vi "attributes-identity-test.vi"(8 "error in (no error)":errorcluster) -> (0 "error out":errorcluster)   [LabVIEW 2013]
uses:
  src/Support/Attribute.Identity/Attribute.Identity.lvclass/Attribute.Identity.ctl
  src/Support/Attribute/Attribute.lvclass/Attribute.ctl
  <vilib>/Utility/LVClass/Get LV Class Name.vi
  <vilib>/addons/_JKI Toolkits/Caraya/classes/Test/Test.lvclass
  <vilib>/addons/_JKI Toolkits/Caraya/classes/Assert/Assert.lvclass
  src/Support/Attribute.Identity/Attribute.Identity.lvclass
  src/Support/Attribute/Attribute.lvclass
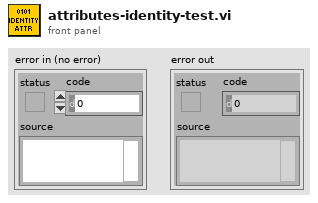
[diagram p1: front panel]
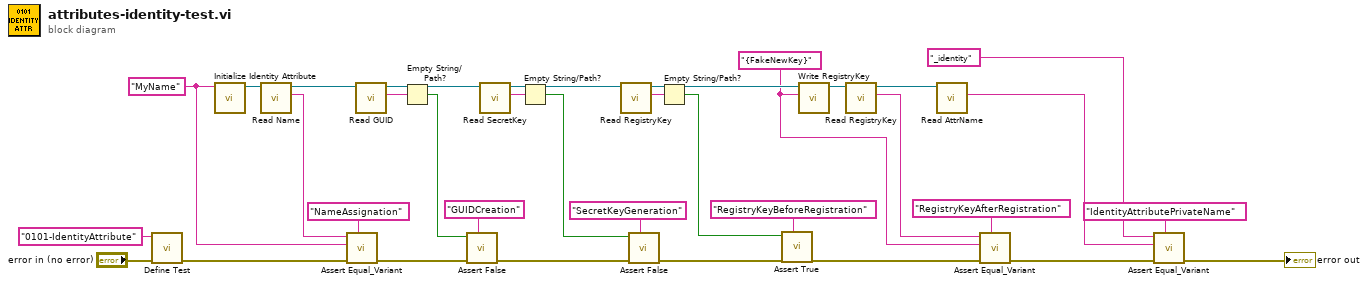
[diagram p0: block diagram]
diagram:
  w8 = "{FakeNewKey}" ("Label (VI Title)")
  w25 = "MyName" ("Name")
  n1 = call <vilib>:"Define Test.vi"("error in (no error)"="error in (no error)", "Label (VI Title)"="0101-IdentityAttribute") -> ("error out"=w33:errorcluster)  [unwired: 9 in]
  n2 = call "Initialize Identity Attribute.vi"("Given Name"=w25) -> ("Attribute.Identity"=w30:refnum<class "Attribute.Identity.lvclass">)  [unwired: 9 in, 1 out]
  n3 = call "Read Name.vi"("Attribute.Identity in"=w30) -> ("Name"=w26:string, "Attribute.Identity out"=w29:refnum<class "Attribute.Identity.lvclass">)  [unwired: 8 in, 1 out]
  n4 = call <vilib>:"Assert Equal_Variant.vi"("Label"="NameAssignation" ("Label (VI Title)"), "error in (no error)"=w33, "Y"=w25, "X"=w26) -> ("error out"=w23:errorcluster)  [unwired: 7 in]
  n5 = call "Read GUID.vi"("Attribute.Identity in"=w29) -> ("GUID"=w24:string, "Attribute.Identity out"=w28:refnum<class "Attribute.Identity.lvclass">)  [unwired: 8 in, 1 out]
  n6 = Empty String/Path?(string/path=w24) -> (empty?=w22:bool)
  n7 = call <vilib>:"Assert False.vi"("Label"="GUIDCreation" ("Label (VI Title)"), "error in (no error)"=w23, "False?"=w22) -> ("error out"=w20:errorcluster)  [unwired: 8 in]
  n8 = call "Read SecretKey.vi"("Attribute.Identity in"=w28) -> ("SecretKey"=w18:string, "Attribute.Identity out"=w16:refnum<class "Attribute.Identity.lvclass">)  [unwired: 8 in, 1 out]
  n9 = Empty String/Path?(string/path=w18) -> (empty?=w17:bool)
  n10 = call "Read RegistryKey.vi"("Attribute.Identity in"=w16) -> ("RegistryKey"=w14:string, "Attribute.Identity out"=w15:refnum<class "Attribute.Identity.lvclass">)  [unwired: 8 in, 1 out]
  n11 = call <vilib>:"Assert False.vi"("Label"="SecretKeyGeneration" ("Label (VI Title)"), "error in (no error)"=w20, "False?"=w17) -> ("error out"=w12:errorcluster)  [unwired: 8 in]
  n12 = Empty String/Path?(string/path=w14) -> (empty?=w11:bool)
  n13 = call <vilib>:"Assert True.vi"("Label"="RegistryKeyBeforeRegistration" ("Label (VI Title)"), "error in (no error)"=w12, "True?"=w11) -> ("error out"=w10:errorcluster)  [unwired: 8 in]
  n14 = call "Write RegistryKey.vi"("RegistryKey"=w8, "Attribute.Identity in"=w15) -> ("Attribute.Identity out"=w27:refnum<class "Attribute.Identity.lvclass">)  [unwired: 8 in, 1 out]
  n15 = call "Read RegistryKey.vi"("Attribute.Identity in"=w27) -> ("RegistryKey"=w9:string, "Attribute.Identity out"=w1:refnum<class "Attribute.Identity.lvclass">)  [unwired: 8 in, 1 out]
  n16 = call "Read AttrName.vi"("Attribute in"=w1) -> ("Attribute Name"=w2:string)  [unwired: 9 in, 1 out]
  n17 = call <vilib>:"Assert Equal_Variant.vi"("Label"="RegistryKeyAfterRegistration" ("Label (VI Title)"), "error in (no error)"=w10, "Y"=w8, "X"=w9) -> ("error out"=w5:errorcluster)  [unwired: 7 in]
  n18 = call <vilib>:"Assert Equal_Variant.vi"("Label"="IdentityAttributePrivateName" ("Label (VI Title)"), "error in (no error)"=w5, "Y"=w2, "X"="_identity" ("Label (VI Title)")) -> ("error out"=→"error out":errorcluster)  [unwired: 7 in]
